vi "Read Shared Variables - SuNLaMP 9216 Slot 2.vi"(9 "channel errors in (no errors)":errorcluster[](array[cluster])) -> (1 "channel errors out":errorcluster[](array[cluster]), 2 "data":dbl[](array[numeric]), 3 "UUIDs":string[](array[string])=["Flow Rate [g/s]", "Density [g/cm^3]", "Return Filter dP [psid]", "Outlet Filter and Flowmeter dp [psid]", "Cooler dP [psid]", "Cooler CO2 In [F]", "Cooler CO2 Out [F]", "Pump Frequency [%]", "Recirc Valve Open [%]"])   [LabVIEW 2020]
uses:
  <vilib>/Utility/error.llb/Error Cluster From Error Code.vi
  <vilib>/ErrorRing/Error Ring.xnode
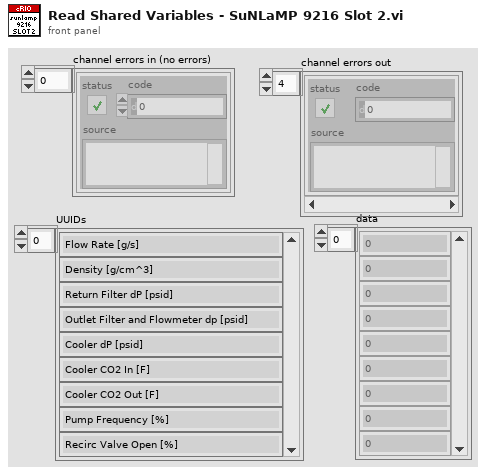
[diagram p1: front panel]
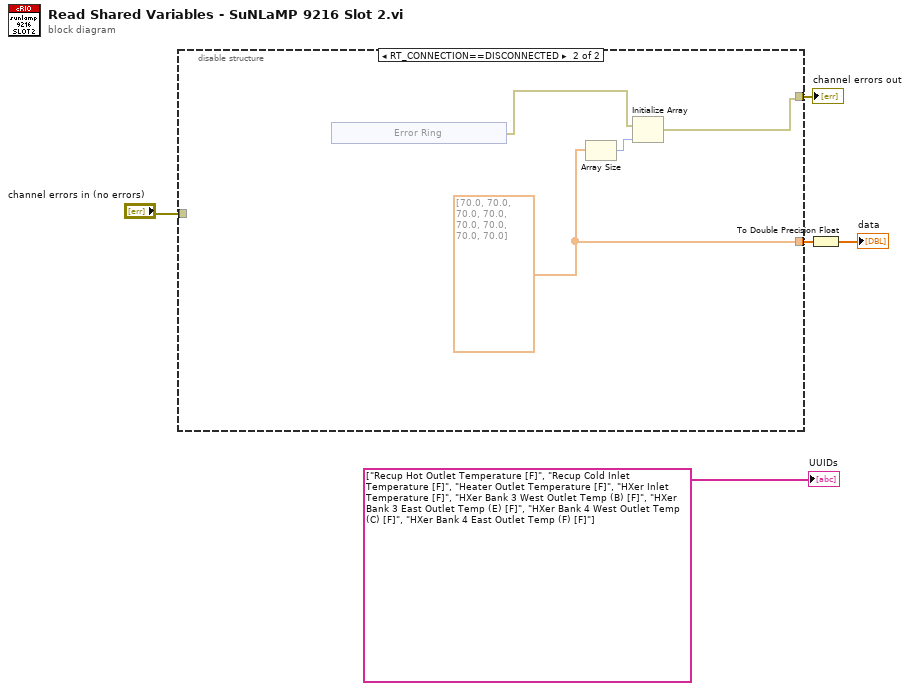
[diagram p0: block diagram]
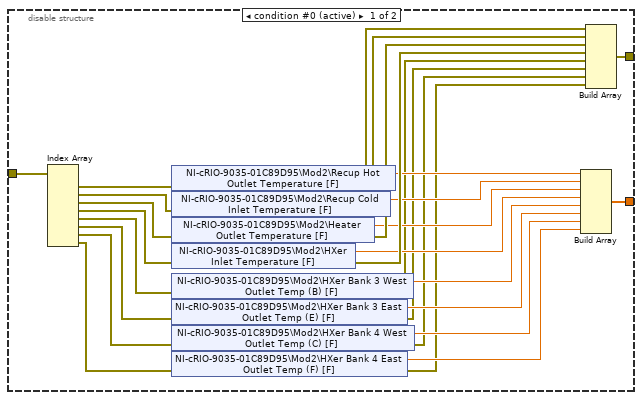
[diagram p2: hidden frame]
diagram:
  n1 = disable-structure shown="RT_CONNECTION==DISCONNECTED" {
    disable-tunnel: [w24 w34] -> w4
    disable-tunnel: "channel errors in (no errors)" -> [w23 _]
    disable-tunnel: [w18 w33] -> w1
    frame condition #0 (active) {
      n2 = Index Array(array=w23) -> (element #1=w22:errorcluster, element #2=w21:errorcluster, element #3=w20:errorcluster, element #4=w19:errorcluster, element #5=w9:errorcluster, element #6=w8:errorcluster, element #7=w7:errorcluster, element #8=w6:errorcluster)  [unwired: 8 in]
      n3 = shared-variable "NI-cRIO-9035-01C89D95\\Mod2\\Recup Hot Outlet Temperature [F]"(error in=w22) -> (w25:dbl, error out=w29:errorcluster)
      n4 = shared-variable "NI-cRIO-9035-01C89D95\\Mod2\\Recup Cold Inlet Temperature [F]"(error in=w21) -> (w26:dbl, error out=w30:errorcluster)
      n5 = shared-variable "NI-cRIO-9035-01C89D95\\Mod2\\Heater Outlet Temperature [F]"(error in=w20) -> (w27:dbl, error out=w31:errorcluster)
      n6 = shared-variable "NI-cRIO-9035-01C89D95\\Mod2\\HXer Inlet Temperature [F]"(error in=w19) -> (w28:dbl, error out=w32:errorcluster)
      n7 = shared-variable "NI-cRIO-9035-01C89D95\\Mod2\\HXer Bank 3 West Outlet Temp (B) [F]"(error in=w9) -> (w17:dbl, error out=w13:errorcluster)
      n8 = shared-variable "NI-cRIO-9035-01C89D95\\Mod2\\HXer Bank 3 East Outlet Temp (E) [F]"(error in=w8) -> (w16:dbl, error out=w12:errorcluster)
      n9 = shared-variable "NI-cRIO-9035-01C89D95\\Mod2\\HXer Bank 4 West Outlet Temp (C) [F]"(error in=w7) -> (w15:dbl, error out=w11:errorcluster)
      n10 = shared-variable "NI-cRIO-9035-01C89D95\\Mod2\\HXer Bank 4 East Outlet Temp (F) [F]"(error in=w6) -> (w14:dbl, error out=w10:errorcluster)
      n11 = Build Array(w25, w26, w27, w28, w17, w16, w15, w14) -> (w18:dbl[])
      n12 = Build Array(w29, w30, w31, w32, w13, w12, w11, w10) -> (w24:errorcluster[])
    }
    frame condition #1 {
      w33 = dbl[] [70.0, 70.0, 70.0, 70.0, 70.0, 70.0, 70.0, 70.0] ("data")
      n13 = xnode "Error Ring"() -> ("error out"=w35:errorcluster)
      n14 = Array Size(array=w33) -> (size(s)=w36:i32)
      n15 = Initialize Array(w35, w36) -> (w34:errorcluster[])
    }
  }
  "channel errors out" <- w4
  n16 = To Double Precision Float(number=w1) -> (double precision float=→"data":dbl[])
  "UUIDs" <- string[] ["Recup Hot Outlet Temperature [F]", "Recup Cold Inlet Temperature [F]", "Heater Outlet Temperature [F]", "HXer Inlet Temperature [F]", "HXer Bank 3 West Outlet Temp (B) [F]", "HXer Bank 3 East Outlet Temp (E) [F]", "HXer Bank 4 West Outlet Temp (C) [F]", "HXer Bank 4 East Outlet Temp (F) [F]"]
